vi "Create.vi"(8 "error in (no error)":errorcluster) -> (0 "error out":errorcluster, 3 "Event Response Handler out":refnum<class "Event Response Handler.lvclass">)   [LabVIEW 2020, in "Event Response Handler.lvclass"]
uses:
  Event Response Handler.lvclass
  Promises/Promise/Promise.lvclass
  Event Response Handler.lvclass/Event Response Handler.ctl
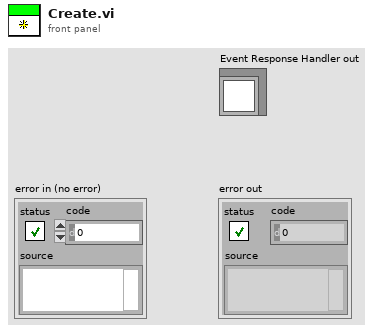
[diagram p1: front panel]
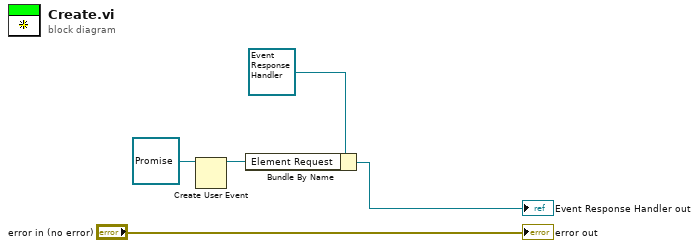
[diagram p0: block diagram]
diagram:
  n1 = Create User Event(user event datatype=refnum<class "Promise.lvclass"> refnum ("Futures:Promise")) -> (user event=w1:refnum<user-event>)  [unwired: 1 in, 1 out]
  n2 = Bundle By Name(cluster=refnum<class "Event Response Handler.lvclass"> refnum ("Event Response Handler in"), "Element Request"=w1) -> (→"Event Response Handler out":refnum<class "Event Response Handler.lvclass">)
  "error out" <- "error in (no error)"
